vi "CThread Find CThread References.vi"(9 "Owning VI":refnum<vi>) -> (0 "error out":errorcluster, 1 "Terminal Set":T1(array[cluster]), 2 "Clone IDs":i16[](array[numeric]), 3 "Paths":path[](array[path]))   [LabVIEW 2012, in "CThread.lvlib"]
uses:
  CThread.lvlib
  <vilib>/Utility/traverseref.llb/TRef TravTarget.ctl
  terminalnode/State.ctl
  <vilib>/Utility/traverseref.llb/VI Scripting - Traverse.lvlib
  terminalnode/CThread VI Terminal Node.xnode
panel:
  in  "error in":errorcluster
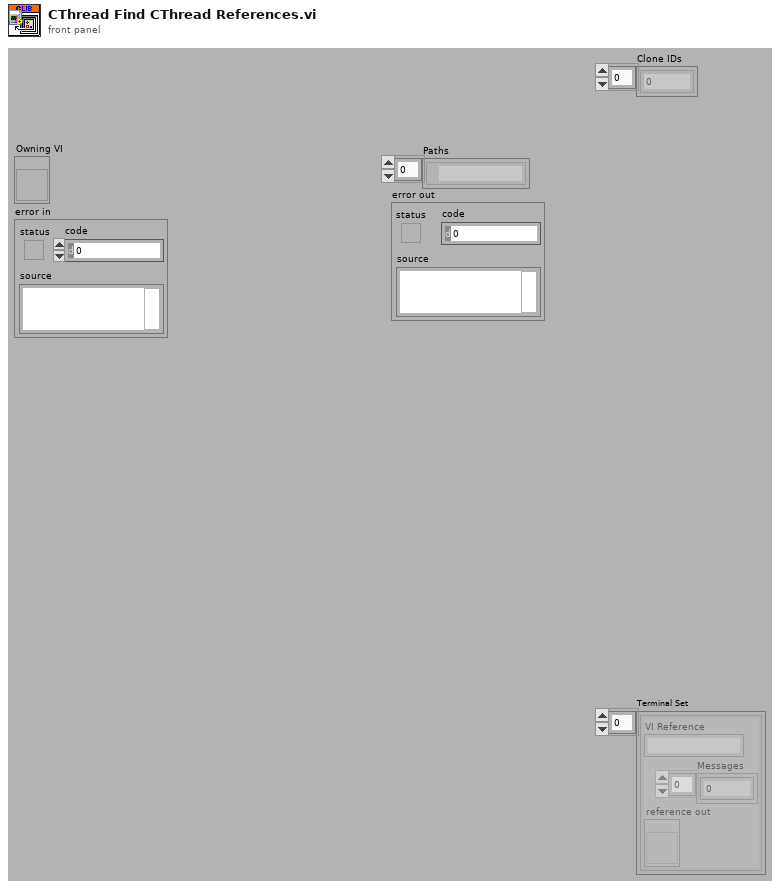
[diagram p1: front panel]
types:
  T1 = cluster{"VI Reference":string, "Messages":u8[], "reference out":refnum<vi>}[]
  T2 = typedef "TRef TravTarget.ctl" = enum16{"FP", "BD", "Other"}
  T3 = typedef "CThread.lvlib/CThread VI Terminal Node.xnode/State.ctl" = cluster{"VI Reference":string, "CLIB VI":string, "Mode":enum16{"TerminalNode", "AdaptorNode"}, "Messages":u8[]}
  T4 = cluster{"Library Version":cluster{"Major":u16, "Minor":u16, "Fix":u16, "Build":u16}, "State":variant}
  T5 = cluster{"VI Reference":string, "Messages":u8[], "reference out":refnum<vi>}
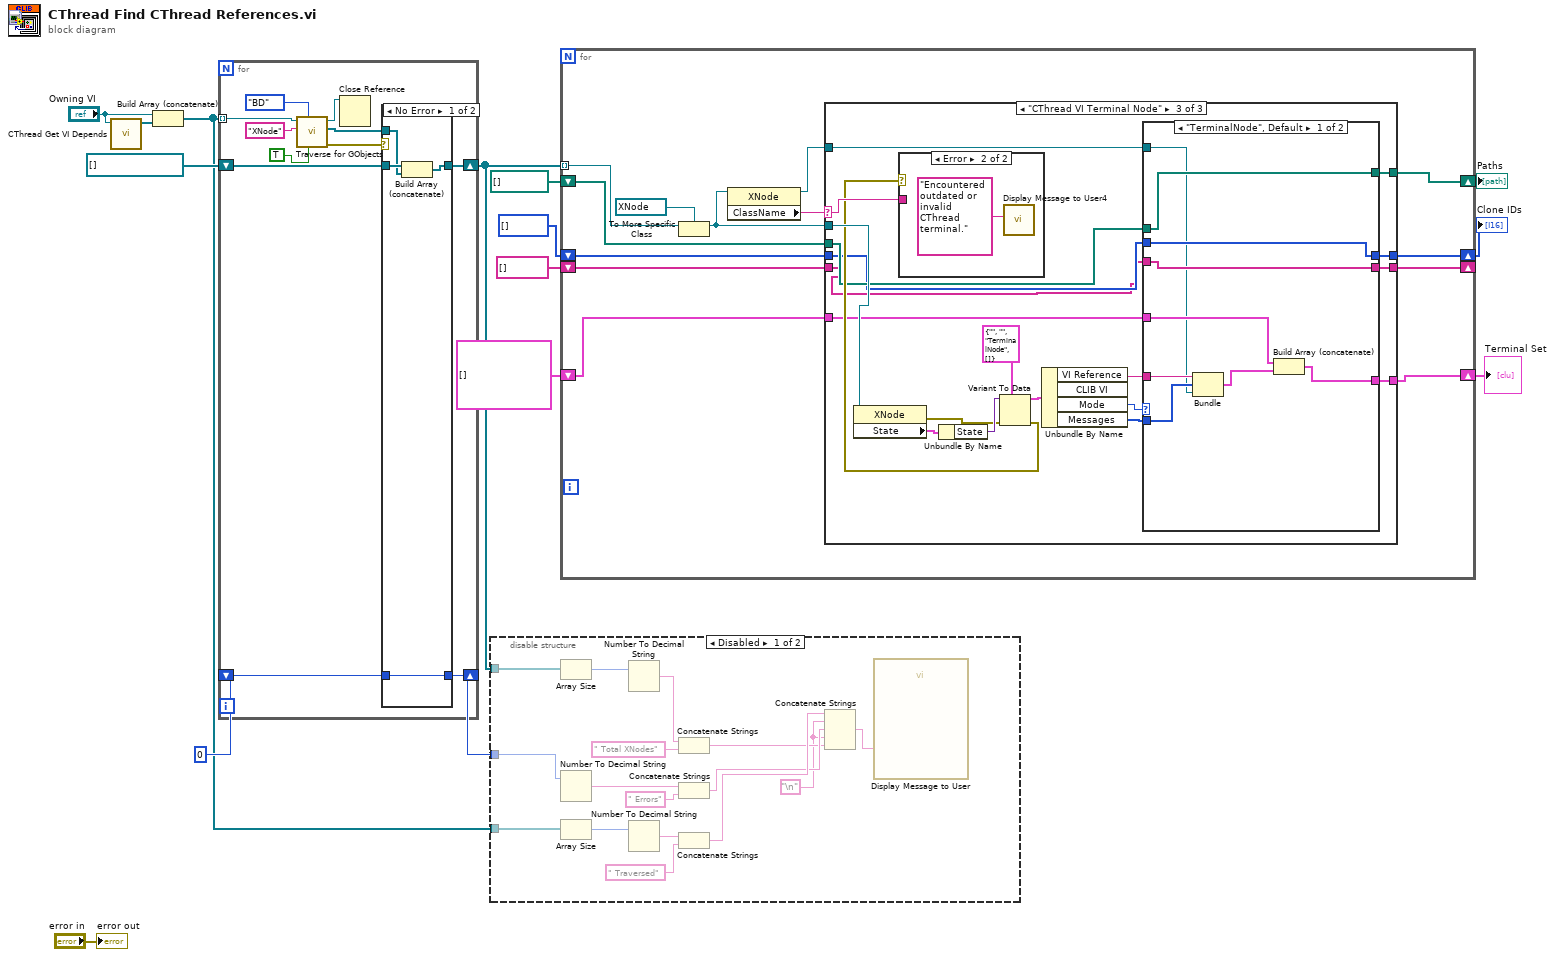
[diagram p0: block diagram]
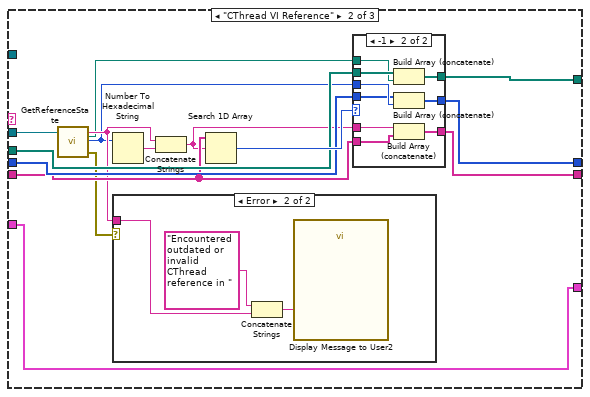
[diagram p4: hidden frame]
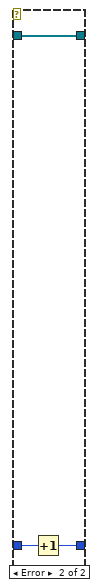
[diagram p9: hidden frame]
diagram:
  n1 = call "CThread Get VI Depends.vi"("Owning VI"="Owning VI") -> ("Array"=w10:refnum<vi>[])  [unwired: 8 in]
  n2 = Build Array (concatenate)("Owning VI", w10) -> (w3:refnum<vi>[])
  n3 = for {
    shift-right: [w26] -> w14
    shift-left: refnum<vi>[] [] -> [w25]
    shift-right: [w23] -> w12
    shift-left: 0 -> [w24]
    tunnel: w3 -> [w22] mode=indexing
    n4 = call <vilib>:"Traverse for GObjects.vi"("Traverse Generated Code (F)"=TRUE, "Traverse Target"=TRef_TravTarget."BD", "Class Name"="XNode", "VI Refnum"=w22) -> ("error out"=w16:errorcluster, "References"=w18:refnum<vi>[], "dup VI Refnum"=w21:refnum<vi>)  [unwired: 4 in, 1 out]
    n5 = Close Reference(reference=w21) -> ()  [unwired: 1 in, 1 out]
    n6 = case shown="No Error" w16 {
      tunnel: w18 -> [w29 _]
      tunnel: [w28 w33] -> w26
      tunnel: w25 -> [w30 w33]
      tunnel: w24 -> [w27 w32]
      tunnel: [w27 w31] -> w23
      frame No Error {
        n7 = Build Array (concatenate)(w30, w29) -> (w28:refnum<vi>[])
      }
      frame Error {
        n8 = Increment(x=w32) -> (x+1=w31:i32)
      }
    }
  }
  n9 = disable-structure shown="Disabled" {
    disable-tunnel: w14 -> [w38 _]
    disable-tunnel: w12 -> [w36 _]
    disable-tunnel: w3 -> [w35 _]
    frame Disabled {
      w39 = "\n"
      n10 = Array Size(array=w38) -> (size(s)=w37:i32)
      n11 = Number To Decimal String(number=w36) -> (decimal integer string=w46:string)  [unwired: 1 in]
      n12 = Array Size(array=w35) -> (size(s)=w34:i32)
      n13 = Number To Decimal String(number=w37) -> (decimal integer string=w42:string)  [unwired: 1 in]
      n14 = Number To Decimal String(number=w34) -> (decimal integer string=w49:string)  [unwired: 1 in]
      n15 = Concatenate Strings(w42, " Total XNodes" ("string")) -> (w40:string)
      n16 = Concatenate Strings(w46, " Errors" ("string")) -> (w44:string)
      n17 = Concatenate Strings(w49, " Traversed" ("string")) -> (w45:string)
      n18 = Concatenate Strings(w45, w39, w44, w39, w40) -> (w43:string)
      n19 = call "Display Message to User"("Message"=w43) -> ()  [unwired: 9 in, 2 out]
    }
    frame Enabled {
    }
  }
  n20 = for {
    tunnel: w14 -> [w61] mode=indexing
    shift-right: [w58] -> _
    shift-left: string[] [] -> [w59]
    shift-right: [w56] -> w7
    shift-left: path[] [] -> [w55]
    shift-right: [w54] -> w4
    shift-left: i16[] [] -> [w53]
    shift-right: [w52] -> w1
    shift-left: T1 [] -> [w51]
    n21 = To More Specific Class(target class=refnum<vi> refnum ("reference out"), reference=w61) -> (specific class reference=w57:refnum<vi>)  [unwired: 1 in, 1 out]
    n22 = property class="XNode"(reference=w57) -> (reference out=w50:refnum<vi>, "ClassName"=w60:string)  [unwired: 1 in, 1 out]
    n23 = case shown="\"CThread VI Terminal Node\"" w60 {
      selector: w60 -> [_ _ w109]
      tunnel: w57 -> [_ w72 w111]
      tunnel: w59 -> [w66 w75 w105]
      tunnel: [w66 w81 w102] -> w58
      tunnel: [w65 w79 w104] -> w56
      tunnel: w55 -> [w65 w76 w107]
      tunnel: [w64 w78 w103] -> w54
      tunnel: w53 -> [w64 w77 w106]
      tunnel: [w63 w67 w99] -> w52
      tunnel: w51 -> [w63 w67 w98]
      tunnel: w50 -> [_ _ w97]
      frame Default {
      }
      frame "CThread VI Reference" {
        n24 = call "GetReferenceState.vi"("CThread Reference"=w72) -> ("VI Name"=w70:string, "VI Path"=w68:path, "Clone"=w69:i16, "error out"=w71:errorcluster)  [unwired: 22 in, 1 out]
        n25 = Number To Hexadecimal String(2:w69) -> (0:w73:string)  [unwired: 1 in]
        n26 = case shown="Error" w71 {
          tunnel: w70 -> [_ w82]
          frame No Error {
          }
          frame Error {
            n27 = Concatenate Strings("Encountered outdated or invalid CThread reference in " ("string"), w82) -> (w84:string)
            n28 = call "Display Message to User2"("Message"=w84) -> ()  [unwired: 9 in, 2 out]
          }
        }
        n29 = Concatenate Strings(w70, w73) -> (w74:string)
        n30 = Search 1D Array(1D array=w75, element=w74) -> (index of element=w80:i32)  [unwired: 1 in]
        n31 = case shown="-1" w80 {
          tunnel: [w85 w96] -> w81
          tunnel: w75 -> [w85 w95]
          tunnel: w68 -> [_ w92]
          tunnel: [w87 w93] -> w79
          tunnel: w76 -> [w87 w94]
          tunnel: [w86 w91] -> w78
          tunnel: w69 -> [_ w90]
          tunnel: w77 -> [w86 w89]
          tunnel: w74 -> [_ w88]
          frame Default {
            # "exists"
          }
          frame -1 {
            n32 = Build Array (concatenate)(w94, w92) -> (w93:path[])
            n33 = Build Array (concatenate)(w89, w90) -> (w91:i16[])
            n34 = Build Array (concatenate)(w88, w95) -> (w96:string[])
          }
        }
      }
      frame "CThread VI Terminal Node" {
        n35 = property class="XNode"(reference=w111) -> (error out=w112:errorcluster, "State"=w116:T4)  [unwired: 1 in, 1 out]
        n36 = Unbundle By Name(w116) -> ("State"=w115:variant)
        n37 = Variant To Data(error in=w112, type=T3 {"VI Reference"="", "CLIB VI"="", "Mode"=enum."TerminalNode", "Messages"=[]} ("State"), Variant=w115) -> (data=w113:T3, error out=w108:errorcluster)
        n38 = case shown="Error" w108 {
          tunnel: w109 -> [_ _]
          frame No Error {
          }
          frame Error {
            n39 = call "Display Message to User4"("Message"="Encountered outdated or invalid CThread terminal." ("string")) -> ()  [unwired: 9 in, 2 out]
          }
        }
        n40 = Unbundle By Name(w113) -> ("VI Reference"=w101:string, "Mode"=w110:enum16{"TerminalNode", "AdaptorNode"}, "Messages"=w100:u8[])  [unwired: 1 out]
        n41 = case shown="\"TerminalNode\", Default" w110 {
          tunnel: w107 -> [w121 w130]
          tunnel: w106 -> [w120 w129]
          tunnel: w105 -> [w119 w128]
          tunnel: [w121 w130] -> w104
          tunnel: [w120 w129] -> w103
          tunnel: [w119 w128] -> w102
          tunnel: w101 -> [w126 _]
          tunnel: w100 -> [w125 _]
          tunnel: [w122 w127] -> w99
          tunnel: w98 -> [w124 w127]
          tunnel: w97 -> [w118 _]
          frame "TerminalNode", Default {
            n42 = Bundle("VI Reference"=w126, "Messages"=w125, "reference out"=w118) -> (w123:T5)  [unwired: 1 in]
            n43 = Build Array (concatenate)(w124, w123) -> (w122:T1)
          }
          frame "AdaptorNode" {
          }
        }
      }
    }
  }
  "Paths" <- w7
  "Clone IDs" <- w4
  "Terminal Set" <- w1
  "error out" <- "error in"
